vi "Anritsu VNA Format Model String.vi"(1 "Model":string) -> (0 "Model":T1=enum."MS20XXX")   [LabVIEW 2011]
uses:
  TypeDefs/Anritsu VNA Model.ctl
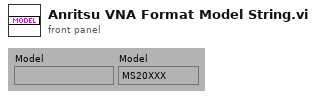
[diagram p1: front panel]
types:
  T1 = typedef "Anritsu VNA Model.ctl" = enum16{"Not Supported", "37XXXX", "MS20XXX", "MS462XX", "MS464XX"}
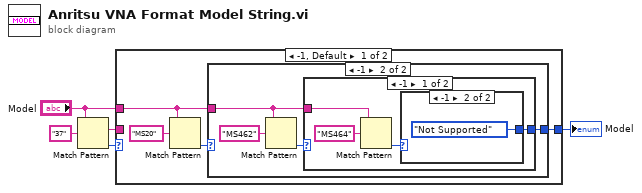
[diagram p0: block diagram]
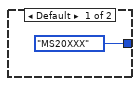
[diagram p2: hidden frame]
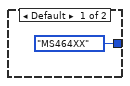
[diagram p3: hidden frame]
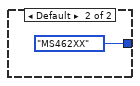
[diagram p4: hidden frame]
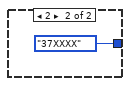
[diagram p5: hidden frame]
diagram:
  n1 = Match Pattern(string="Model", regular expression="37") -> (match substring=w2:string, offset past match=w3:i32)  [unwired: 3 out]
  n2 = case shown="-1, Default" w3 {
    tunnel: [w6 Anritsu_VNA_Model."37XXXX" ("Model")] -> w5
    tunnel: "Model" -> [w7 _]
    tunnel: w2 -> [_ _]
    frame -1, Default {
      n3 = Match Pattern(string=w7, regular expression="MS20") -> (offset past match=w8:i32)  [unwired: 4 out]
      n4 = case shown="-1" w8 {
        tunnel: w7 -> [_ w11]
        tunnel: [Anritsu_VNA_Model."MS20XXX" ("Model") w12] -> w6
        frame Default {
        }
        frame -1 {
          n5 = Match Pattern(string=w11, regular expression="MS462") -> (offset past match=w13:i32)  [unwired: 4 out]
          n6 = case shown="-1" w13 {
            tunnel: [w18 Anritsu_VNA_Model."MS462XX" ("Model")] -> w12
            tunnel: w11 -> [w16 _]
            frame -1 {
              n7 = Match Pattern(string=w16, regular expression="MS464") -> (offset past match=w15:i32)  [unwired: 4 out]
              n8 = case shown="-1" w15 {
                tunnel: [Anritsu_VNA_Model."MS464XX" ("Model") Anritsu_VNA_Model."Not Supported" ("Model")] -> w18
                frame Default {
                }
                frame -1 {
                }
              }
            }
            frame Default {
            }
          }
        }
      }
    }
    frame 2 {
    }
  }
  "Model" <- w5
